vi "StreamChansEventTest.vi"() -> ()   [LabVIEW 2017]
panel:
  in  "termchar":u8=4
  in  "stop":bool
  in  "VISA resource name":refnum<visa-resource-name>
  out "error out":errorcluster
  out "ChanStrReturned":string
  in  "error in (no error)":errorcluster
  in  "Amplifier Chans":i32[](listbox)=[1, 4, 13, 14, 15, 16, 17, 22]
  in  "Update Channels":bool
  in  "Accel/Vbat":i32[](listbox)
  out "ChanSelect(uint32)":u32[](array[numeric])
  out "ChanSelString":string
  in  "update stream chans (Teensy char)":string="h"
  out "setChansResponse1":string
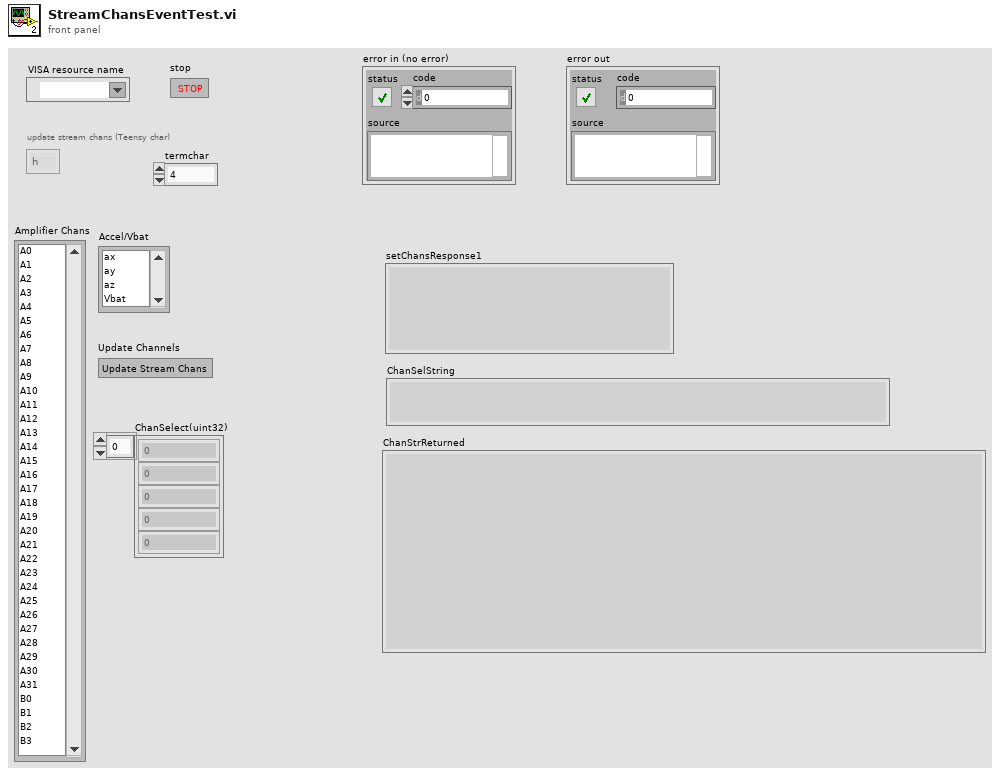
[diagram p1: front panel]
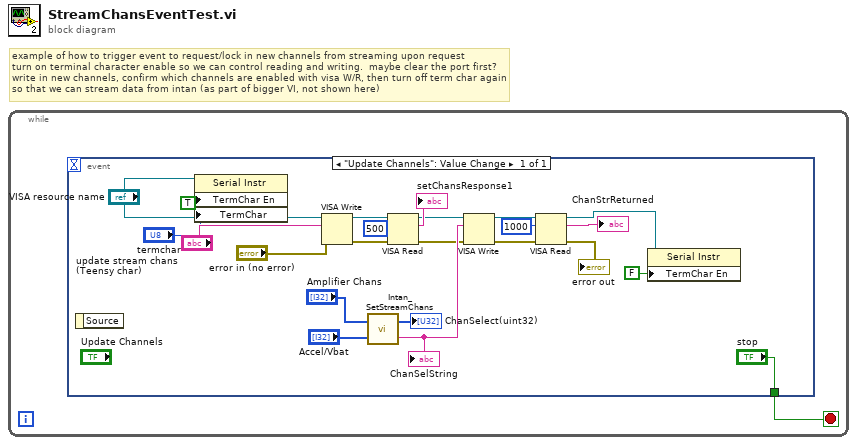
[diagram p0: block diagram]
diagram:
  # "example of how to trigger event to request/lock in new channels from streaming upon request\nturn on terminal character enable so we can control reading and writing.  maybe clear the port first?  \nwrite in new channels, confirm which channels are enabled with visa W/R, then turn off term char again\nso that we can stream data from intan (as part of bigger VI, not shown here)"
  n1 = while {
    stop <- w1 stop-if-true
    n2 = event shown="[0] \"Update Channels\": Value Change" {
      selector: _ -> [_]
      dyn-events: _ -> [_]
      timeout: _ -> [_]
      tunnel: ["stop"] -> w1
      event "Update Channels": Value Change {
        n3 = event-data() -> ()  [unwired: 1 in, 1 out]
        n4 = property class="Serial Instr"(reference="VISA resource name", "TermChar En"=TRUE ("Message Based Settings:Termination Character Enable"), "TermChar"="termchar") -> ()  [unwired: 1 in, 2 out]
        n5 = VISA Write(VISA resource name="VISA resource name", write buffer="update stream chans (Teensy char)", error in (no error)="error in (no error)") -> (VISA resource name out=w21:refnum<visa-resource-name>, error out=w15:errorcluster)  [unwired: 1 out]
        n6 = call "Intan_SetStreamChans.vi"("Accel/Vbat"="Accel/Vbat", "Amplifier Chans"="Amplifier Chans") -> ("ChanSelString"=w17:string, "ChanSelect(uint32)"=→"ChanSelect(uint32)":u32[])
        "ChanSelString" <- w17
        n7 = VISA Read(VISA resource name=w21, byte count=u32 500, error in (no error)=w15) -> (VISA resource name out=w16:refnum<visa-resource-name>, read buffer=→"setChansResponse1":string, error out=w13:errorcluster)  [unwired: 1 out]
        n8 = VISA Write(VISA resource name=w16, write buffer=w17, error in (no error)=w13) -> (VISA resource name out=w12:refnum<visa-resource-name>, error out=w11:errorcluster)  [unwired: 1 out]
        n9 = VISA Read(VISA resource name=w12, byte count=u32 1000, error in (no error)=w11) -> (VISA resource name out=w6:refnum<visa-resource-name>, read buffer=→"ChanStrReturned":string, error out=→"error out":errorcluster)  [unwired: 1 out]
        n10 = property class="Serial Instr"(reference=w6, "TermChar En"=FALSE ("Message Based Settings:Termination Character Enable")) -> ()  [unwired: 1 in, 2 out]
      }
    }
  }
